vi "SetPathInZip.vi"(1 "TempFolderPath":path, 2 "FilePath":path) -> (0 "PathInZip":path)   [LabVIEW 2013]
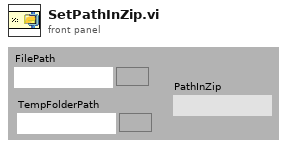
[diagram p1: front panel]
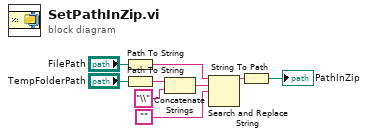
[diagram p0: block diagram]
diagram:
  n1 = Path To String(path="FilePath") -> (string=w6:string)
  n2 = Path To String(path="TempFolderPath") -> (string=w3:string)
  n3 = Concatenate Strings(w3, "\\" ("string")) -> (w1:string)
  n4 = Search and Replace String(input string=w6, search string=w1, replace string="") -> (result string=w4:string)  [unwired: 5 in, 3 out]
  n5 = String To Path(string=w4) -> (path=→"PathInZip":path)
